vi "UDP-ImgSender.vi"() -> ()   [LabVIEW 2020]
doc: "Uses DataSocket to write array data. This example works for writing the data to the DataSocket Server (for live data). \n \nThe Writer, Server, and Reader can all be on the same computer or different computers. The Writer and Reader URLs should point to the computer where the DataSocket Server is."
panel:
  out "Image":T1(plugin-control)
  in  "Stop":bool
  # "UDP - Image Sender"
  # "Instruction:\n1. Run UDP Sender;\n2. Run Image Receiver.\n3. see the images transfered\n to image reveiver."
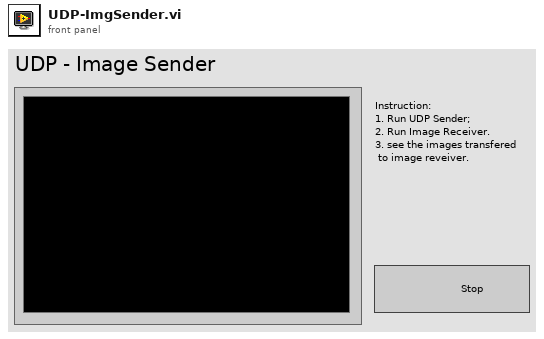
[diagram p1: front panel]
types:
  T1 = typedef "IMAQ Image.ctl" = refnum<image>
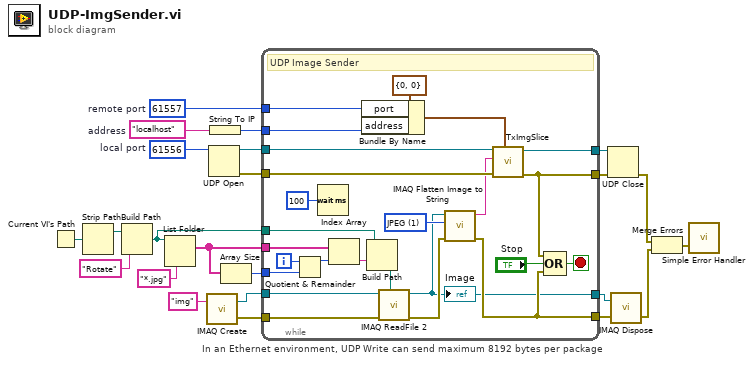
[diagram p0: block diagram]
diagram:
  w6 = "localhost"  # address
  w7 = u16 61557  # remote port
  w9 = u16 61556  # local port
  # "In an Ethernet environment, UDP Write can send maximum 8192 bytes per package"
  n1 = Current VI's Path() -> (path=w20:path)
  n2 = Strip Path(path=w20) -> (stripped path=w19:path)  [unwired: 1 out]
  n3 = Build Path(base path=w19, name or relative path="Rotate") -> (appended path=w14:path)
  n4 = List Folder(path=w14, pattern="*.jpg") -> (filenames=w12:string[])  [unwired: 2 in, 3 out]
  n5 = call "IMAQ Create"("Image Name"="img") -> ("New Image"=w15:T1, "error out"=w16:errorcluster)  [unwired: 4 in]
  n6 = UDP Open(11:w9) -> (port=w2:refnum<k16>, 0:w8:errorcluster)  [unwired: 4 in, 1 out]
  n7 = String To IP(1:w6) -> (0:w5:u32)
  n8 = Array Size(array=w12) -> (size(s)=w13:i32)
  n9 = while {
    tunnel: [w35] -> w22
    tunnel: [w33] -> w21
    tunnel: w16 -> [w45]
    tunnel: w15 -> [w44]
    tunnel: w14 -> [w43]
    tunnel: w12 -> [w39]
    tunnel: w13 -> [w38]
    tunnel: w8 -> [w32]
    tunnel: w7 -> [w27]
    tunnel: w5 -> [w26]
    tunnel: [w31] -> w4
    tunnel: w2 -> [w30]
    tunnel: [w29] -> w1
    i -> [w40]
    stop <- w36 stop-if-true
    w47 = 1 items=["None", "JPEG", "PACKED BINARY"] ("Compression (None)")
    # "UDP Image Sender"
    n10 = Quotient & Remainder(x=w40, y=w38) -> (x-y*floor(x/y)=w41:i32)  [unwired: 1 out]
    n11 = Wait (ms)(milliseconds to wait=u32 100) -> ()  [unwired: 1 out]
    n12 = Index Array(array=w39, index=w41) -> (element=w37:string)
    n13 = Bundle By Name(cluster=cluster{"address":u32, "port":u16} {"address"=0, "port"=0} ("address"), "port"=w27, "address"=w26) -> (w24:cluster{"address":u32, "port":u16})
    n14 = Build Path(base path=w43, name or relative path=w37) -> (appended path=w42:path)
    n15 = call "IMAQ ReadFile 2"("File Path"=w42, "error in (no error)"=w45, "Image"=w44) -> ("error out"=w46:errorcluster, "Image Out"=w33:T1)  [unwired: 4 in, 3 out]
    "Image" <- w33
    n16 = call "IMAQ Flatten Image to String"("error in (no error)"=w46, "Compression (None)"=w47, "Image"=w33) -> ("error out"=w35:errorcluster, "Data String"=w28:string)  [unwired: 7 in]
    n17 = call "TxImgSlice.vi"("address"=w24, "error in"=w32, "DataString"=w28, "Conn"=w30) -> ("error out"=w31:errorcluster, "Conn"=w29:refnum<k16>)  [unwired: 6 in]
    n18 = Compound Arithmetic op=OR(w31, "Stop", w35) -> (w36:bool)
  }
  n19 = UDP Close(connection ID=w1, 8:w4) -> (error out=w3:errorcluster)  [unwired: 1 out]
  n20 = call "IMAQ Dispose"("Image"=w21, "error in (no error)"=w22) -> ("error out"=w11:errorcluster)  [unwired: 4 in]
  n21 = Merge Errors(w3, w11) -> (w10:errorcluster)
  n22 = call <vilib>:"Simple Error Handler.vi"("error in (no error)"=w10) -> ()  [unwired: 4 in, 5 out]
